vi "Get FPGA Data Refs.vi"(8 "error in":errorcluster, 9 "Device Ref in":T2 format="%.0x", 11 "Item Ref in":T2 format="%.0x") -> (0 "error out":errorcluster, 1 "Output Data":dbl[](array[numeric]), 2 "Output Block Data Refs":T5[](array[typedef]) {"Data Reference" format="%.0x"}, 3 "Item Ref out":T2=18446744073709551615 format="%.0x", 4 "Input Data":dbl[](array[numeric]), 5 "To FPGA":T1[](array[typedef]) {"VS ref" format="%.0x"}, 6 "Input Block Data Refs":T5[](array[typedef]) {"Data Reference" format="%.0x"}, 7 "From FPGA":T1[](array[typedef]) {"VS ref" format="%.0x"})   [LabVIEW 2016, in "Scan Engine Custom Device.lvlib"]
uses:
  Scan Engine Custom Device.lvlib
  <vilib>/NI Veristand/Custom Device API/Block Data Reference.ctl
  <vilib>/NI Veristand/Custom Device API/Data Reference.ctl
  <vilib>/NI Veristand/Custom Device API/Custom Device Item Ref.ctl
  Type Defs/UDV Data.ctl
  Type Defs/UDV Data Type.ctl
  Type Defs/FXP Config.ctl
  <vilib>/NI Veristand/Custom Device API/Data Access Type.ctl
  <vilib>/NI Veristand/Custom Device API/Custom Device Channel Type.ctl
  <vilib>/NI Veristand/Custom Device API/Custom Device API.lvlib
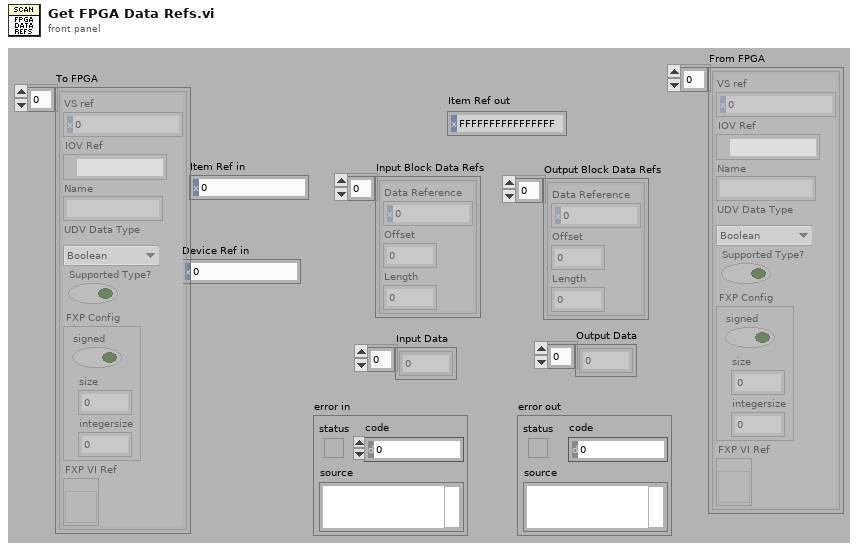
[diagram p1: front panel]
types:
  T1 = typedef "Scan Engine Custom Device.lvlib/UDV Data.ctl" = cluster{"VS ref":T2, "IOV Ref":refnum<k21>, "Name":string, "UDV Data Type":T3, "Supported Type?":bool, "FXP Config":T4, "FXP VI Ref":refnum<vi>}
  T2 = typedef "Custom Device API.lvlib/Custom Device Item Ref.ctl" = u64
  T3 = typedef "Scan Engine Custom Device.lvlib/UDV Data Type.ctl" = enum16{"Boolean", "Fixed Point", "Int8", "Int16", "Int32", "Int64", "U32 Bit Field", "UInt8", "UInt16", "UInt32", "UInt64", "Other"}
  T4 = typedef "Scan Engine Custom Device.lvlib/FXP Config.ctl" = cluster{"signed":bool, "size":u32, "integersize":i32}
  T5 = typedef "Custom Device API.lvlib/Block Data Reference.ctl" = cluster{"Data Reference":T6, "Offset":u64, "Length":u64}
  T6 = typedef "Custom Device API.lvlib/Data Reference.ctl" = i32
  T7 = typedef "Custom Device API.lvlib/Data Access Type.ctl" = enum16{"Read", "Write"}
  T8 = typedef "Custom Device API.lvlib/Custom Device Channel Type.ctl" = enum16{"Input", "Output"}
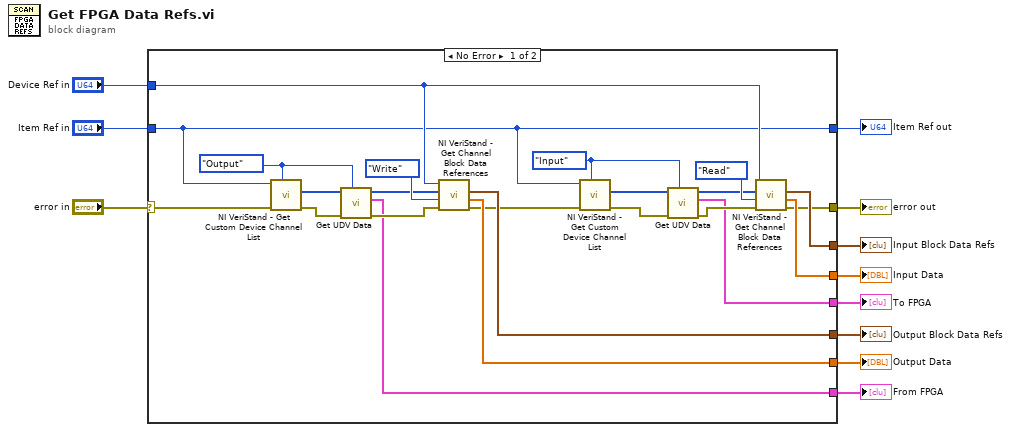
[diagram p0: block diagram]
diagram:
  n1 = case shown="No Error" "error in" {
    selector: "error in" -> [w20 w36]
    tunnel: [w34 _] -> w11
    tunnel: [w33 _] -> w10
    tunnel: [w32 _] -> w9
    tunnel: [w31 _] -> w8
    tunnel: "Device Ref in" -> [w28 _]
    tunnel: [w25 _] -> w6
    tunnel: [w22 _] -> w5
    tunnel: [w21 w36] -> w4
    tunnel: "Item Ref in" -> [w13 w35]
    tunnel: [w13 w35] -> w1
    frame No Error {
      w12 = Custom_Device_Channel_Type."Input" ("Channel Type")
      w17 = Custom_Device_Channel_Type."Output" ("Channel Type")
      n2 = call <vilib>:"NI VeriStand - Get Custom Device Channel List.vi"("Channel Type"=w17, "error in (no error)"=w20, "Device Ref in"=w13) -> ("error out"=w19:errorcluster, "Specified Channel Ref List"=w18:T2[])  [unwired: 7 out]
      n3 = call "Get UDV Data.vi"("Channel Type"=w17, "error in (no error)"=w19, "Channel Ref List in"=w18) -> ("error out"=w23:errorcluster, "UDV Data"=w22:T1[], "Channel Ref List out"=w24:T2[])  [unwired: 6 in]
      n4 = call <vilib>:"NI VeriStand - Get Channel Block Data References.vi"("error in (no error)"=w23, "Access"=Data_Access_Type."Write", "Channel Refs"=w24, "Device Ref in"=w28) -> ("error out"=w16:errorcluster, "Values Array"=w34:dbl[], "Block Data Refs"=w33:T5[])  [unwired: 4 in, 1 out]
      n5 = call <vilib>:"NI VeriStand - Get Custom Device Channel List.vi"("Channel Type"=w12, "error in (no error)"=w16, "Device Ref in"=w13) -> ("error out"=w15:errorcluster, "Specified Channel Ref List"=w14:T2[])  [unwired: 7 out]
      n6 = call "Get UDV Data.vi"("Channel Type"=w12, "error in (no error)"=w15, "Channel Ref List in"=w14) -> ("error out"=w26:errorcluster, "UDV Data"=w25:T1[], "Channel Ref List out"=w27:T2[])  [unwired: 6 in]
      n7 = call <vilib>:"NI VeriStand - Get Channel Block Data References.vi"("error in (no error)"=w26, "Access"=Data_Access_Type."Read", "Channel Refs"=w27, "Device Ref in"=w28) -> ("error out"=w21:errorcluster, "Values Array"=w31:dbl[], "Block Data Refs"=w32:T5[])  [unwired: 4 in, 1 out]
    }
    frame Error {
    }
  }
  "error out" <- w4
  "Item Ref out" <- w1
  "Output Data" <- w11
  "Output Block Data Refs" <- w10
  "Input Data" <- w8
  "Input Block Data Refs" <- w9
  "From FPGA" <- w5
  "To FPGA" <- w6
